vi "View_Results_File.vi"() -> ()   [LabVIEW 2010]
uses:
  Anemometry Sub Vis/Globals/Meas_global.vi
panel:
  out "?":string[][](table)
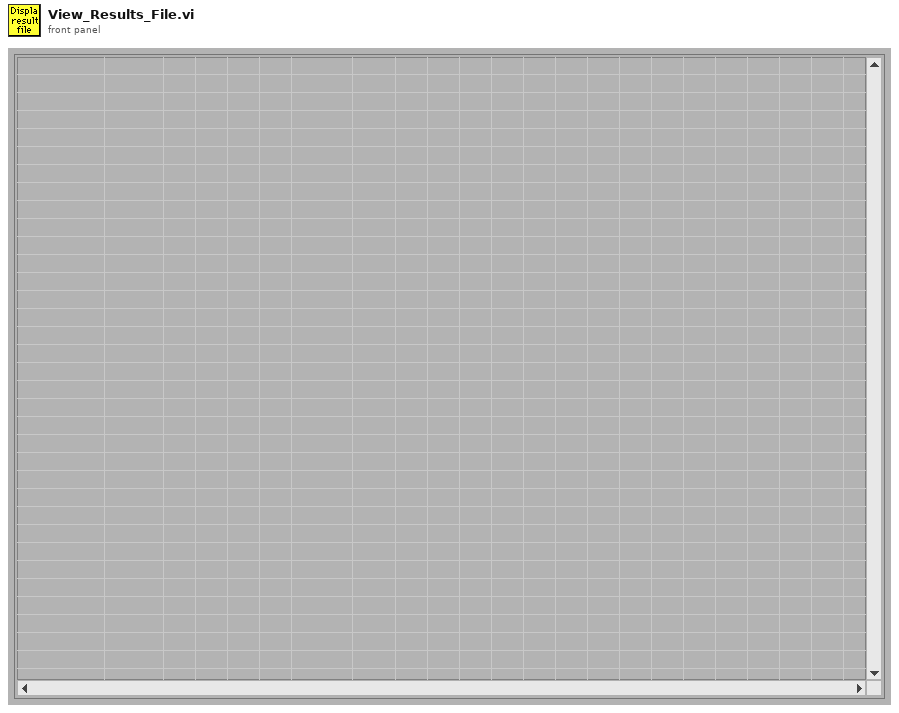
[diagram p1: front panel]
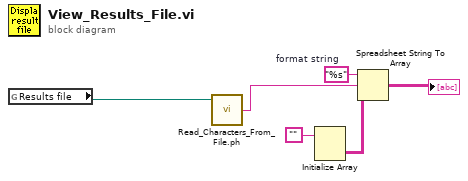
[diagram p0: block diagram]
diagram:
  w3 = "%s"  # format string
  n1 = global read "Meas_global.vi" "Results file"() -> (w1:path)
  n2 = call "Read_Characters_From_File.ph.vi"("file path (dialog if empty)"=w1) -> ("character string"=w2:string)  [unwired: 5 in, 3 out]
  n3 = Initialize Array("") -> (w5:string[][])  [unwired: 2 in]
  n4 = Spreadsheet String To Array(format string=w3, spreadsheet string=w2, array type (2D Dbl)=w5) -> (array=→"?":string[][])  [unwired: 1 in]
